vi "Get Current User.vi"(8 "error in (no error)":errorcluster) -> (0 "error out":errorcluster, 3 "current user":string)   [LabVIEW 2017, in "Windows Security.lvlib"]
doc: "Returns the current (logged in) user."
uses:
  Windows Security.lvlib
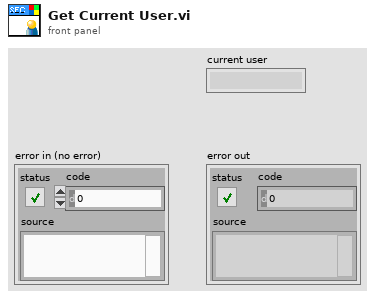
[diagram p1: front panel]
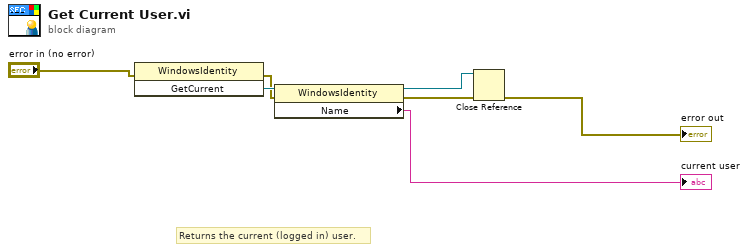
[diagram p0: block diagram]
diagram:
  # "Returns the current (logged in) user."
  n1 = invoke class="WindowsIdentity" method="GetCurrent"(error in="error in (no error)") -> (error out=w5:errorcluster, "GetCurrent"=w7:refnum<k24>)  [unwired: 2 in, 1 out]
  n2 = property class="WindowsIdentity"(reference=w7, error in=w5) -> (reference out=w1:refnum<k24>, error out=w4:errorcluster, "Name"=→"current user":string)
  n3 = Close Reference(reference=w1, error in (no error)=w4) -> (error out=→"error out":errorcluster)
